vi "reconCluster.vi"(7 "Array 6":bool[](array[boolean]), 8 "Variable header":string[](array[string]), 9 "Alias":string[](array[string]), 10 "Data in":string[][](array[string]), 11 "variant in":variant) -> (1 "time":u32, 3 "variant out":variant)   [LabVIEW 2013]
uses:
  <vilib>/vision/Image Controls.llb/IMAQ Image.ctl
  <vilib>/vision/NI_Vision_Development_Module.lvlib
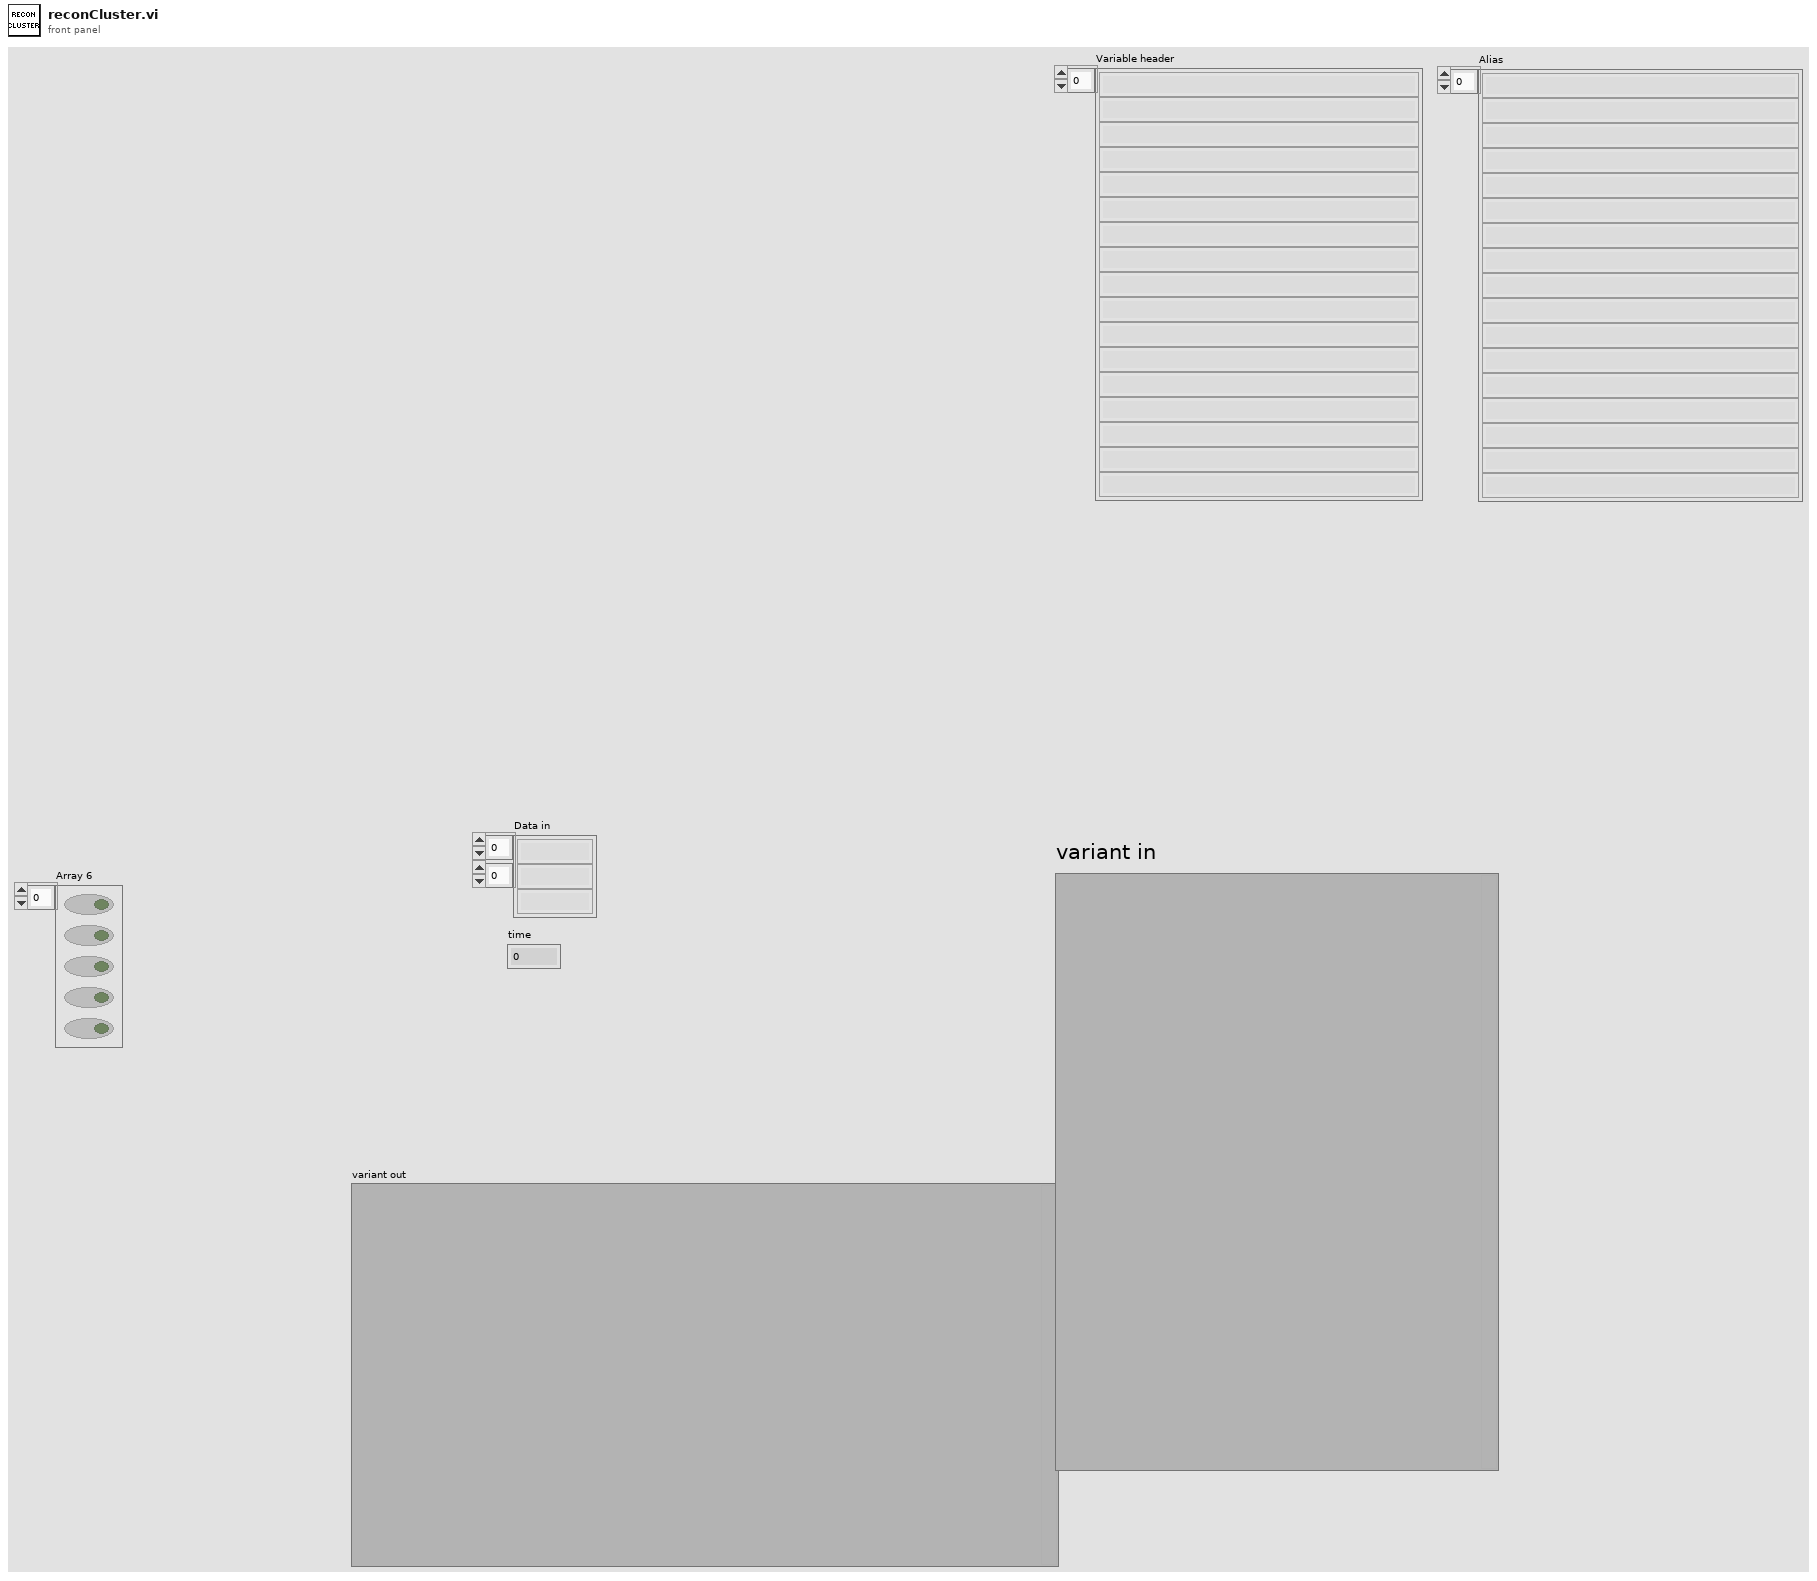
[diagram p1: front panel]
types:
  T1 = typedef "IMAQ Image.ctl" = refnum<image>
  T2 = typedef "Type Descriptor Enumeration__ogtk.ctl" = enum8{"<Null>", "I8", "I16", "I32", "I64", "U8", "U16", "U32", "U64", "SGL", "DBL", "EXT", "CSG", "CDB", "CXT", "0x0F", "0x10", "0x11", "0x12", "0x13", "0x14", "Enum U8", "Enum U16", "Enum U32", "Enum U64", "SGL PQ", "DBL PQ", "EXT PQ", "CSG PQ", "CDB PQ", "CXT PQ", "0x1F", "0x20", "Boolean", "0x22", "0x23", "0x24", "0x25", "0x26", "0x27", "0x28", "0x29", "0x2A", "0x2B", "0x2C", "0x2D", "0x2E", "0x2F", "String", "0x31", "Path", "Pict", "0x34", "0x35", "0x36", "DAQ", "0x38", "0x39", "0x3A", "0x3B", "0x3C", "0x3D", "0x3E", "0x3F", "Array", "0x41", "0x42", "0x43", "0x44", "0x45", "0x46", "0x47", "0x48", "0x49", "0x4A", "0x4B", "0x4C", "0x4D", "0x4E", "0x4F", "Cluster", "0x51", "0x52", "Variant", "Waveform", "0x55", "0x56", "0x57", "0x58", "0x59", "0x5A", "0x5B", "0x5C", "0x5D", "0x5E", "0x5F", "0x60", "0x61", "0x62", "0x63", "0x64", "0x65", "0x66", "0x67", "0x68", "0x69", "0x6A", "0x6B", "0x6C", "0x6D", "0x6E", "0x6F", "Refnum"}
  T3 = typedef "Image Type" = u32
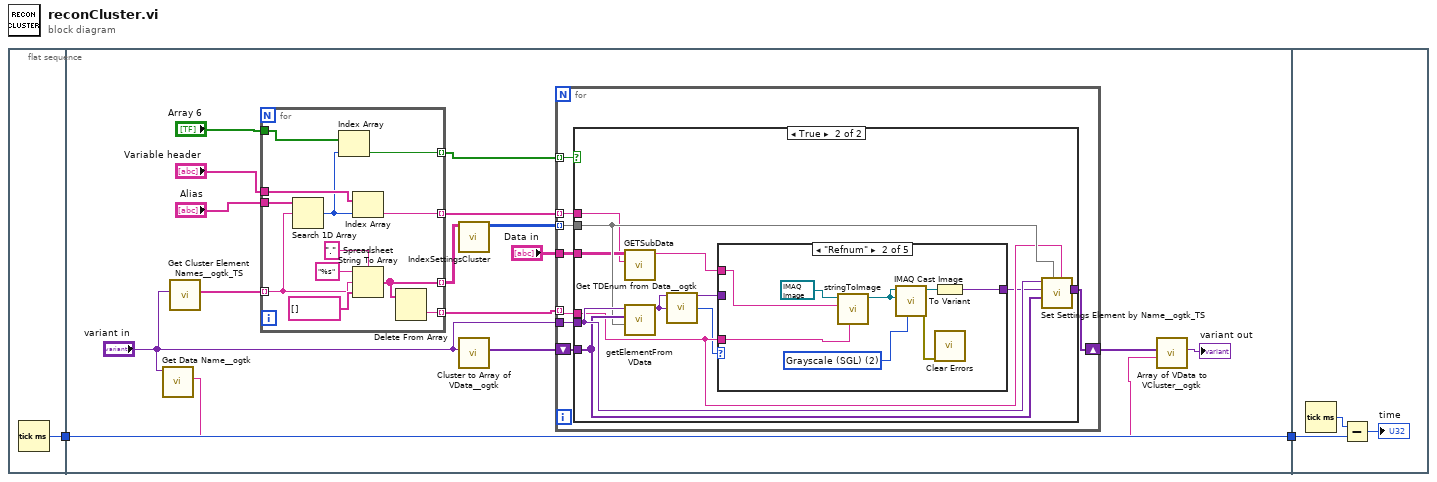
[diagram p0: block diagram]
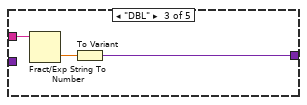
[diagram p4: hidden frame]
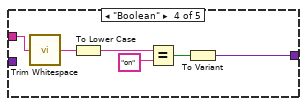
[diagram p5: hidden frame]
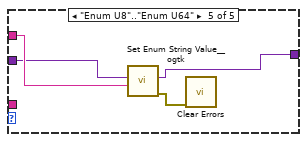
[diagram p6: hidden frame]
diagram:
  n1 = flat-sequence {
    tunnel: [w3] -> w2
    tunnel: w2 -> [w12]
    tunnel: [w12] -> w1
    tunnel: w1 -> [w75]
    frame #0 {
      n2 = Tick Count (ms)() -> (millisecond timer value=w3:u32)
    }
    frame #1 {
      n3 = call <userlib>:"Get Data Name__ogtk.vi"("Data"="variant in") -> ("Data Name"=w6:string)  [unwired: 8 in, 2 out]
      n4 = call "Get Cluster Element Names__ogtk_TS.vi"("Variant"="variant in") -> ("Names (Array)"=w18:string[])  [unwired: 9 in, 1 out]
      n5 = for {
        tunnel: w18 -> [w67] mode=indexing
        tunnel: [w70] -> w19 mode=indexing
        tunnel: [w69] -> w15 mode=indexing
        tunnel: "Alias" -> [w68]
        tunnel: "Variable header" -> [w66]
        tunnel: [w65] -> w8 mode=indexing
        tunnel: "Array 6" -> [w64]
        tunnel: [w62] -> w4 mode=indexing
        n6 = Search 1D Array(1D array=w68, element=w67) -> (index of element=w63:i32)  [unwired: 1 in]
        n7 = Index Array(array=w64, index=w63) -> (element=w62:bool)
        n8 = Index Array(array=w66, index=w63) -> (element=w65:string)
        n9 = Spreadsheet String To Array(delimiter (Tab)=".", format string="%s", spreadsheet string=w67, array type (2D Dbl)=string[] []) -> (array=w70:string[])
        n10 = Delete From Array(array=w70) -> (deleted portion=w69:string)  [unwired: 2 in, 1 out]
      }
      n11 = call "IndexSettingsCluster.vi"("Names Array"=w19) -> ("index Array"=w16:i32[][])  [unwired: 10 in]
      n12 = call <userlib>:"Cluster to Array of VData__ogtk.vi"("Cluster"="variant in") -> ("Array of VData"=w17:variant[])  [unwired: 9 in, 1 out]
      n13 = for {
        shift-right: [w27] -> w14
        shift-left: w17 -> [w25]
        tunnel: w16 -> [w24] mode=indexing
        tunnel: "variant in" -> [w26]
        tunnel: w15 -> [w21] mode=indexing
        tunnel: "Data in" -> [w23]
        tunnel: w8 -> [w22] mode=indexing
        tunnel: w4 -> [w20] mode=indexing
        n14 = case shown="True" w20 {
          tunnel: [w28 w39] -> w27
          tunnel: w26 -> [_ w38]
          tunnel: w25 -> [w28 w37]
          tunnel: w24 -> [_ w36]
          tunnel: w23 -> [_ w35]
          tunnel: w22 -> [_ w34]
          tunnel: w21 -> [_ w32]
          frame False {
          }
          frame True {
            n15 = call "GETSubData.vi"("Variable Header"=w34, "Data out"=w35) -> ("delimiter (Tab)"=w33:string)  [unwired: 9 in]
            n16 = call "getElementFromVData.vi"("index Array 2"=w36, "Settings VData"=w37, "Cluster in"=w38) -> ("element out"=w29:variant)  [unwired: 6 in, 2 out]
            n17 = call <userlib>:"Get TDEnum from Data__ogtk.vi"("Data"=w29) -> ("Type Descriptor Enumeration"=w31:T2)  [unwired: 4 in]
            n18 = case shown="\"Refnum\"" w31 {
              tunnel: w33 -> [_ w48 w51 w57 w61]
              tunnel: w32 -> [_ w42 _ _ _]
              tunnel: [w40 w43 w49 w52 w59] -> w30
              tunnel: w29 -> [w40 _ _ _ w60]
              frame "<Null>", Default {
              }
              frame "Refnum" {
                w46 = T3 2 items=["Grayscale (U8)", "Grayscale (I16)", "Grayscale (SGL)", "Complex (CSG)", "RGB (U32)", "HSL (U32)", "RGB (U64)", "Grayscale (U16)"] ("Image Type")
                n19 = call "stringToImage.vi"("label text (image name)"=w42, "data in"=w48, "Refnum in"=T1 refnum ("Image")) -> ("Refnum out"=w47:T1)  [unwired: 6 in, 2 out]
                n20 = call "IMAQ Cast Image"("Image Type"=w46, "Image Dst"=w47, "Image Src"=w47) -> ("error out"=w41:errorcluster, "Image Dst Out"=w44:T1)  [unwired: 7 in]
                n21 = To Variant(anything=w44) -> (Variant=w43:variant)
                n22 = call <vilib>:"Clear Errors.vi"("error in (no error)"=w41) -> ()  [unwired: 6 in, 1 out]
              }
              frame "DBL" {
                n23 = Fract/Exp String To Number(string=w51) -> (number=w50:dbl)  [unwired: 3 in, 1 out]
                n24 = To Variant(anything=w50) -> (Variant=w49:variant)
              }
              frame "Boolean" {
                n25 = call <vilib>:"Trim Whitespace.vi"("string"=w57) -> ("trimmed string"=w56:string)  [unwired: 1 in]
                n26 = To Lower Case(string=w56) -> (all lower case string=w55:string)
                n27 = Equal?(x=w55, y="on" ("x")) -> (x = y?=w53:bool)
                n28 = To Variant(anything=w53) -> (Variant=w52:variant)
              }
              frame "Enum U8".."Enum U64" {
                n29 = call <userlib>:"Set Enum String Value__ogtk.vi"("String Value"=w61, "Default Enum Value"=w60) -> ("error out"=w58:errorcluster, "Enum"=w59:variant)  [unwired: 8 in]
                n30 = call <vilib>:"Clear Errors.vi"("error in (no error)"=w58) -> ()  [unwired: 6 in, 1 out]
              }
            }
            n31 = call "Set Settings Element by Name__ogtk_TS.vi"("element Name"=w32, "index Array"=w36, "Settings VData"=w37, "New Element Value"=w30, "Cluster"=w38) -> ("Settings VData out"=w39:variant[])  [unwired: 5 in, 1 out]
          }
        }
      }
      n32 = call <userlib>:"Array of VData to VCluster__ogtk.vi"("Cluster Name"=w6, "Array"=w14) -> ("VCluster"=→"variant out":variant)  [unwired: 8 in, 1 out]
    }
    frame #2 {
      n33 = Tick Count (ms)() -> (millisecond timer value=w76:u32)
      n34 = Subtract(x=w76, y=w75) -> (x-y=→"time":u32)
    }
  }
